vi "GlobalHowAmI.vi"() -> ()   [LabVIEW 2012]
panel:
  out "HowAmI?":cluster{"T":dbl, "Battery":dbl, "Temp":dbl}
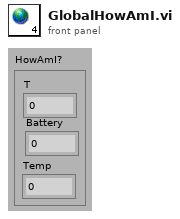
[diagram p1: front panel]
diagram:
